vi "compare_doubles.vi"(1 "range":dbl=1e-15, 2 "y":dbl, 3 "x":dbl) -> (0 "equal / in range?":bool)   [LabVIEW 2021]
doc: "This VI compares two numbers (doubles) and checks if they are with a certain range.\nThe default range is set to 1 femto = 1E-15."
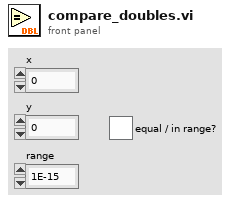
[diagram p1: front panel]
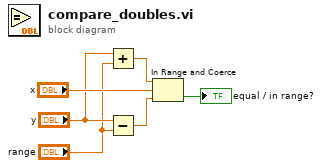
[diagram p0: block diagram]
diagram:
  n1 = Add(x="y", y="range") -> (x+y=w5:dbl)
  n2 = Subtract(x="y", y="range") -> (x-y=w4:dbl)
  n3 = In Range and Coerce(upper limit=w5, x="x", lower limit=w4) -> (In Range?=→"equal / in range?":bool)  [unwired: 1 out]
